vi "Autonomous Delay.vi"   [LabVIEW 2017]
types:
  T1 = typedef "WPI_AnalogChannelDevRef.ctl" = cluster{"DevStatus":errorcluster, "Analog Channel":T2}
  T2 = typedef "FPGA_AIChannel.ctl" = enum8{"AI 0", "AI 1", "AI 2", "AI 3", "AI MXP 0", "AI MXP 1", "AI MXP 2", "AI MXP 3", "Invalid"}
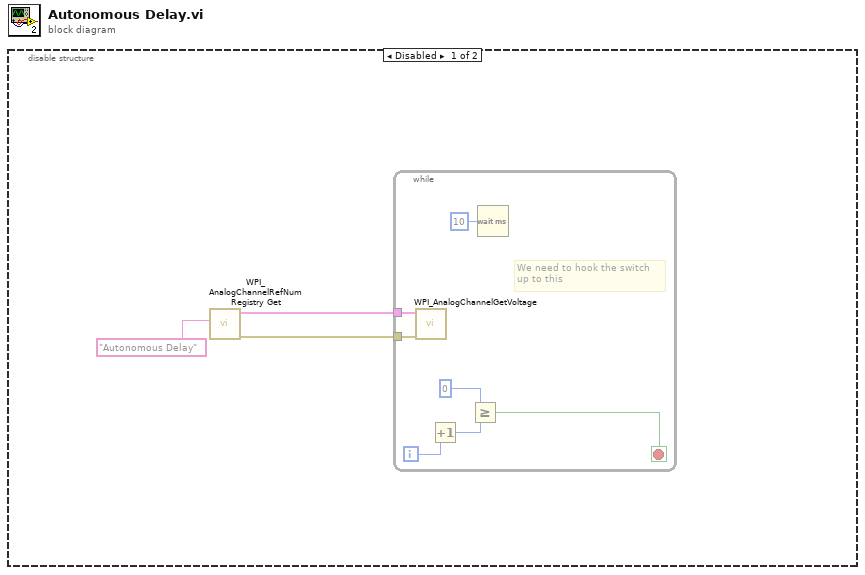
[diagram p0: block diagram]
diagram:
  n1 = disable-structure shown="Disabled" {
    frame Disabled {
      n2 = call <vilib>:"WPI_AnalogChannelRefNum Registry Get.vi"("refnum name"="Autonomous Delay") -> ("error out"=w2:errorcluster, "AIDeviceRef"=w1:T1)  [unwired: 9 in]
      n3 = while {
        tunnel: w2 -> [w5]
        tunnel: w1 -> [w4]
        i -> [w9]
        stop <- w10 stop-if-true
        # "We need to hook the switch\nup to this"
        n4 = call <vilib>:"WPI_AnalogChannelGetVoltage.vi"("error in (no error)"=w5, "AIDeviceRef"=w4) -> ()  [unwired: 7 in, 3 out]
        n5 = Increment(x=w9) -> (x+1=w8:i32)
        n6 = Greater Or Equal?(x=w8, y=0) -> (x >= y?=w10:bool)
        n7 = Wait (ms)(milliseconds to wait=u32 10) -> ()  [unwired: 1 out]
      }
    }
    frame Enabled {
    }
  }
